vi "Subvi DO.vi"(2 "DO":refnum<k21>="Connector1/DIO0", 8 "AsyncTrigger":bool, 10 "FIFO":refnum<k21>="DB0") -> ()   [LabVIEW 2017]
uses:
  <vilib>/rvi/Emulation/niFpgaGetClockAttributes.vi
  <vilib>/rvi/Emulation/niFpgaSctlEmulationGetInTimedLoop.vi
  <vilib>/rvi/Emulation/niFpgaEmulationReportErrorSimple.vi
  GV preframeclock.vi
  <vilib>/rvi/Emulation/niFpgaCriticalErrorInLSC.vi
  GV DOdelay_tick.vi
  GV FIFOINtimeout_tick.vi
  <vilib>/rvi/eio/common/nirviEmuTemplateMethod_errors.vi
  <vilib>/rvi/DataTransferAndStorage/Container/Common/niFpgaContainerExecOnDevCompGetState.vi
  <vilib>/rvi/Emulation/niFpgaEmulationIsFPGAContextNoSignature.vi
  <vilib>/rvi/errors/niFpgaSetErrorForExecOnDevCompSimple.vi
  <vilib>/rvi/eio/common/nirviEmuReportErrorAndStop.vi
  <vilib>/rvi/DataTransferAndStorage/Container/Common/niFpgaContainerGetUniqueNameForEmu.vi
  <vilib>/rvi/FIFO/Fifo_Resource/nirvififoEmulationSetSize.vi
  <vilib>/rvi/FIFO/Fifo_Resource/nirviFifoEmulationQueueMgr.vi
  <instcachedir>/0/nirviFifoEmulationQueueMgr_E5CAEC123FF24DC58D834DCA3CDAA9B5.lvgen/nirviFifoEmulationQueueMgr_E5CAEC123FF24DC58D834DCA3CDAA9B5_001.vi
  <vilib>/rvi/FIFO/Fifo_Resource/nirvififoEmulationDetermineInputValidOut.vi
  <vilib>/rvi/FIFO/Fifo_Resource/nirvififoEmulationCreateLock.vi
  <vilib>/rvi/Emulation/niFpgaProcessEmulError.vi
  <vilib>/rvi/FIFO/Fifo_Resource/nirvififoEmulationObtainLock.vi
  <vilib>/rvi/FIFO/Fifo_Resource/nirvififoEmulationReleaseLock.vi
  <vilib>/rvi/occurrence/nirviWaitOnOccurrenceBase.vi
  <vilib>/rvi/errors/nirviReportUnexpectedCaseInternalError.vi
  <vilib>/rvi/errors/nirviReportUnexpectedCaseInternalError (U32).vi
  <vilib>/Utility/error.llb/Clear Errors.vi
  <vilib>/rvi/interface/RandomDataEmulation/niFpgaRandomDataHandleErrors.vi
  <vilib>/eio/EIONode/EIONode.xnode
  <vilib>/rvi/DataTransferAndStorage/Container/XNode/niFpgaContainer.xnode
  <vilib>/rvi/FIFO/Fifo_Resource/niFpgaFifoEmulationRefIn.vi
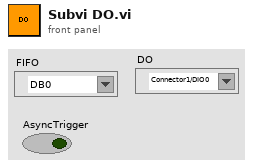
[diagram p1: front panel]
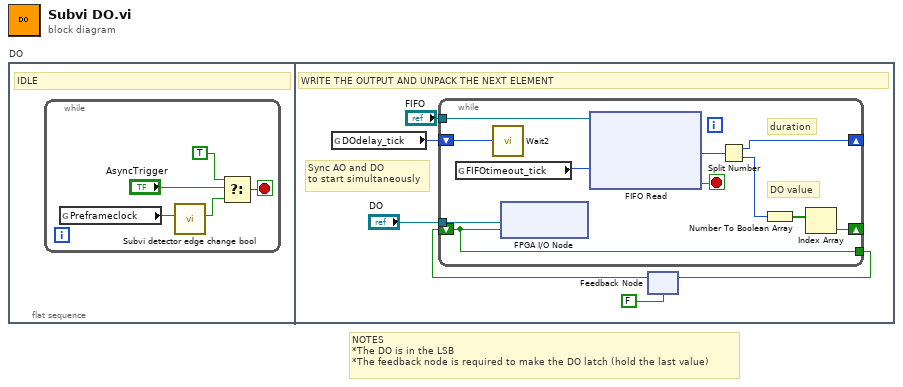
[diagram p0: block diagram]
diagram:
  # "NOTES\n*The DO is in the LSB\n*The feedback node is required to make the DO latch (hold the last value)"
  n1 = flat-sequence "DO" {
    frame #0 {
      # "IDLE"
      n2 = while {
        stop <- w4 stop-if-true
        n3 = global read "GV Preframeclock.vi" "Preframeclock"() -> (w1:bool)
        n4 = call "Subvi detector edge change bool.vi"("Input"=w1) -> ("Output"=w2:bool)  [unwired: 8 in]
        n5 = Select(t=TRUE, s="AsyncTrigger", f=w2) -> (s? t:f=w4:bool)
      }
    }
    frame #1 {
      # "Sync AO and DO\nto start simultaneously"
      # "WRITE THE OUTPUT AND UNPACK THE NEXT ELEMENT"
      n6 = global read "GV DOdelay_tick.vi" "DOdelay_tick"() -> (w7:u32)
      n7 = feedback #1(FALSE) -> (w10:bool)
      n8 = while {
        shift-right: [w18] -> _
        shift-left: w10 -> [w12]
        shift-right: [w20] -> _
        shift-left: w7 -> [w19]
        tunnel: [w12] -> w9
        tunnel: "FIFO" -> [w14]
        tunnel: "DO" -> [w13]
        stop <- w16 stop-if-true
        # "DO value"
        # "duration"
        n9 = global read "GV FIFOINtimeout_tick.vi" "FIFOtimeout_tick"() -> (w15:i32)
        n10 = call "Wait2"("Count(Ticks)"=w19) -> ()  [unwired: 1 out]
        n11 = xnode "FPGA I/O Node"("I/O Item"=w12, "FPGA I/O In"=w13) -> ()  [unwired: 1 out]
        n12 = xnode ("FIFO Read")("Timeout"=w15, "FIFO In"=w14) -> ("Element"=w17:u32, "Timed Out?"=w16:bool)  [unwired: 1 out]
        n13 = Split Number(x=w17) -> (hi(x)=w20:u16, lo(x)=w21:u16)
        n14 = Number To Boolean Array(number=w21) -> (Boolean array=w22:bool[])
        n15 = Index Array(array=w22) -> (element=w18:bool)  [unwired: 1 in]
      }
      n16 = feedback-in #1(w9) -> ()
    }
  }
